vi "Get Cols Information.vi"(7 "Table Name":string, 8 "error in (no error)":errorcluster, 11 "LV-ORM in":refnum<class "LV-ORM.lvclass">) -> (0 "error out":errorcluster, 1 "Table Name 2":string, 2 "columns data type":string[](array[string]), 3 "LV-ORM out":refnum<class "LV-ORM.lvclass">, 4 "column names":string[](array[string]))   [LabVIEW 2018, in "LV-ORM.lvclass"]
uses:
  LV-ORM.lvclass
  LV-ORM.lvclass/LV-ORM.ctl
  Serializer/Serializer.lvclass
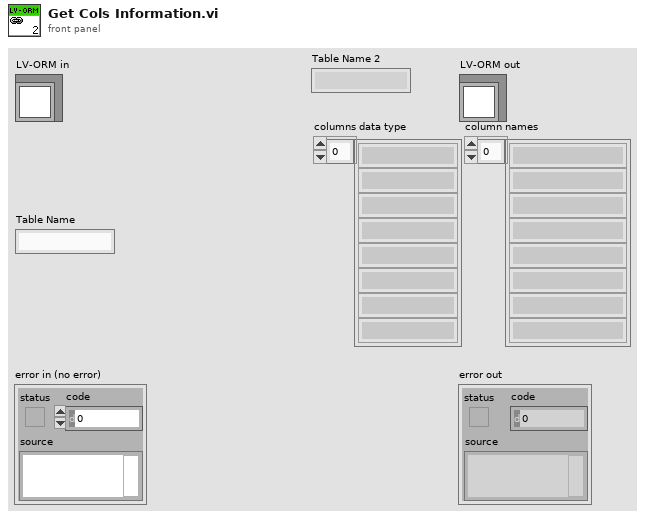
[diagram p1: front panel]
types:
  T1 = typedef "NI_Database_API.lvlib/Conn ObjectReference.ctl" = refnum<k1>
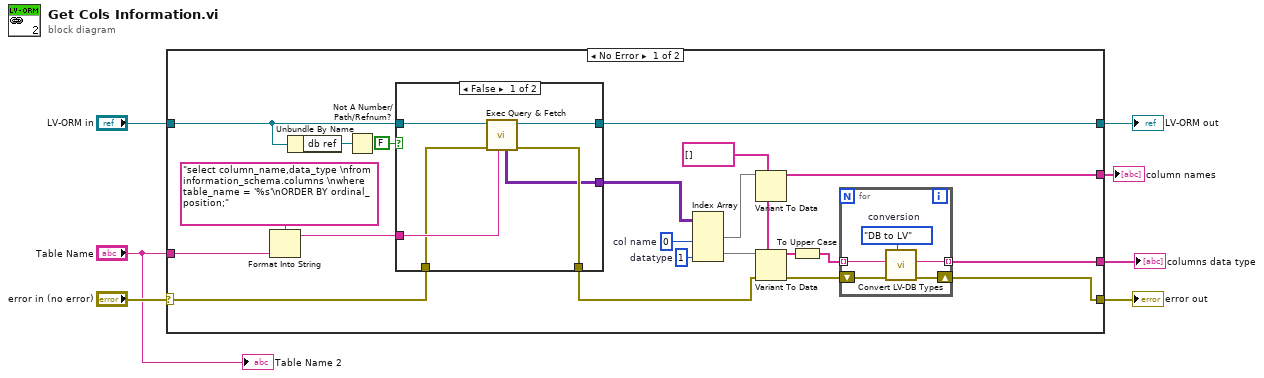
[diagram p0: block diagram]
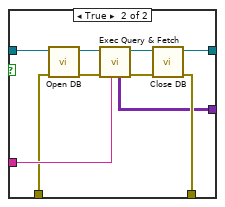
[diagram p2: hidden frame]
diagram:
  n1 = case shown="No Error" "error in (no error)" {
    selector: "error in (no error)" -> [w22 w51]
    tunnel: [w13 w51] -> w6
    tunnel: [w23 w50] -> w4
    tunnel: "LV-ORM in" -> [w25 w50]
    tunnel: "Table Name" -> [w27 _]
    tunnel: [w14 _] -> w2
    tunnel: [w8 _] -> w1
    frame No Error {
      w10 = string[] []
      w12 = 0  # col name
      w18 = 1  # datatype
      n2 = Format Into String(format string="select column_name,data_type \nfrom information_schema.columns \nwhere table_name = '%s'\nORDER BY ordinal_position;", w27) -> (resulting string=w24:string)  [unwired: 2 in, 1 out]
      n3 = Unbundle By Name(w25) -> ("db ref"=w26:T1)
      n4 = Not A Number/Path/Refnum?(number/path/refnum=w26) -> ()  [unwired: 1 out]
      n5 = case shown="False" FALSE {
        tunnel: w25 -> [w39 w49]
        tunnel: w24 -> [w38 w47]
        tunnel: [w37 w43] -> w23
        tunnel: w22 -> [w36 w42]
        tunnel: [w35 w41] -> w16
        tunnel: [w34 w40] -> w17
        frame False {
          n6 = call "Exec Query & Fetch.vi"("scripts"=w38, "error in"=w36, "orm in"=w39) -> ("error out"=w35:errorcluster, "orm out"=w37:refnum<class "LV-ORM.lvclass">, "recordset data"=w34:variant[][])  [unwired: 6 in]
        }
        frame True {
          n7 = call "Open DB.vi"("error in (no error)"=w42, "LV-ORM in"=w49) -> ("error out"=w46:errorcluster, "LV-ORM out"=w48:refnum<class "LV-ORM.lvclass">)  [unwired: 8 in]
          n8 = call "Exec Query & Fetch.vi"("scripts"=w47, "error in"=w46, "orm in"=w48) -> ("error out"=w45:errorcluster, "orm out"=w44:refnum<class "LV-ORM.lvclass">, "recordset data"=w40:variant[][])  [unwired: 6 in]
          n9 = call "Close DB.vi"("error in"=w45, "LV-ORM in"=w44) -> ("error out"=w41:errorcluster, "LV-ORM out"=w43:refnum<class "LV-ORM.lvclass">)  [unwired: 8 in]
        }
      }
      n10 = Index Array(array=w17, index (col) #1=w12, index (col) #2=w18) -> (element #1=w11:variant[], element #2=w19:variant[])  [unwired: 2 in]
      n11 = Variant To Data(type=w10, Variant=w11) -> (data=w8:string[])  [unwired: 1 in, 1 out]
      n12 = Variant To Data(error in=w16, type=w10, Variant=w19) -> (data=w20:string[], error out=w15:errorcluster)
      n13 = To Upper Case(1:w20) -> (0:w21:string[])
      n14 = for {
        tunnel: [w32] -> w14 mode=indexing
        tunnel: w21 -> [w31] mode=indexing
        shift-right: [w29] -> w13
        shift-left: w15 -> [w30]
        w33 = enum16{"LV to DB", "DB to LV"}."DB to LV"  # conversion
        n15 = call "Convert LV-DB Types.vi"("conversion"=w33, "error in"=w30, "DataType"=w31) -> ("error out"=w29:errorcluster, "Converted Type"=w32:string)  [unwired: 7 in]
      }
    }
    frame Error {
    }
  }
  "error out" <- w6
  "LV-ORM out" <- w4
  "columns data type" <- w2
  "column names" <- w1
  "Table Name 2" <- "Table Name"
